vi "enable_channels.vi"(5 "channel":i32[](array[numeric]), 6 "celay":i32[](array[numeric]), 7 "vclip":i32[](array[numeric]), 8 "error in":errorcluster, 9 "vatt":i32[](array[numeric]), 10 "id_in":i32, 11 "connection ID":refnum<k5>) -> (0 "error out":errorcluster, 1 "id_out":i32, 3 "connection ID out":refnum<k5>)   [LabVIEW 2009]
doc: "This VI sends a command to the Integration Board and provides the received data when necessary."
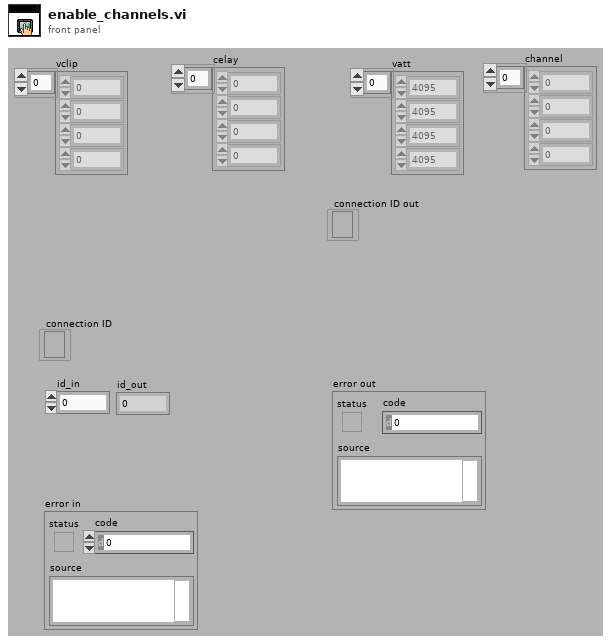
[diagram p1: front panel]
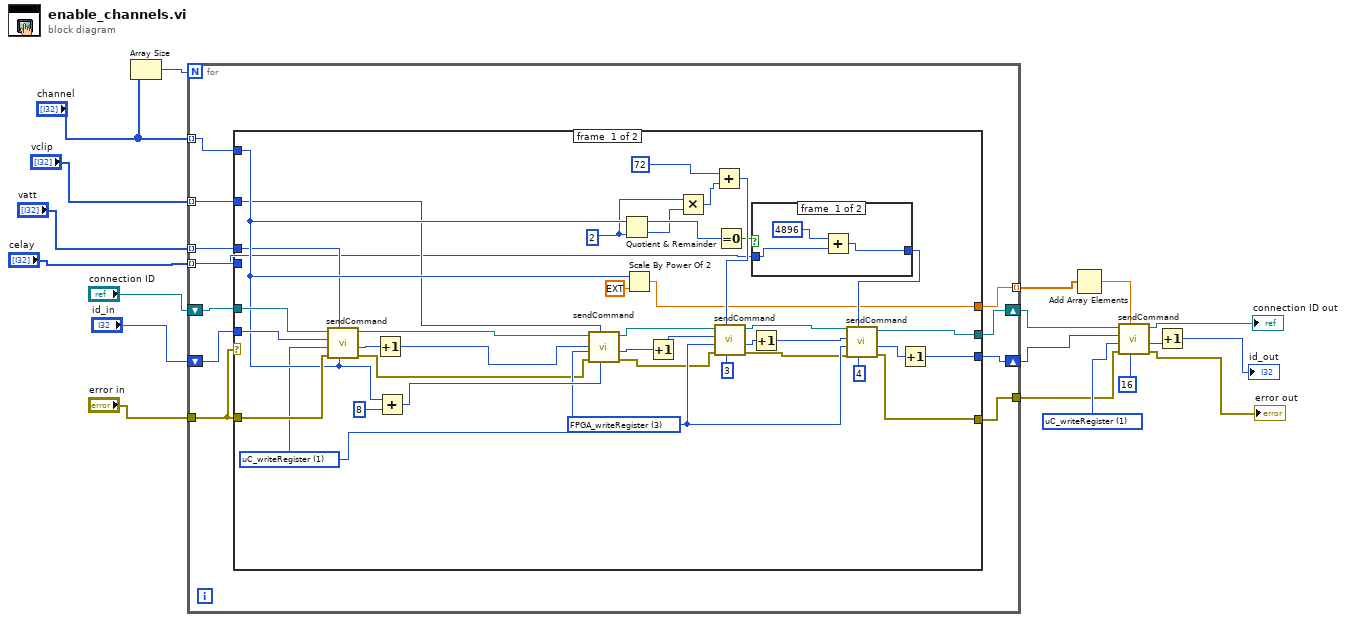
[diagram p0: block diagram]
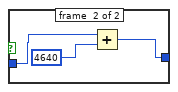
[diagram p2: hidden frame]
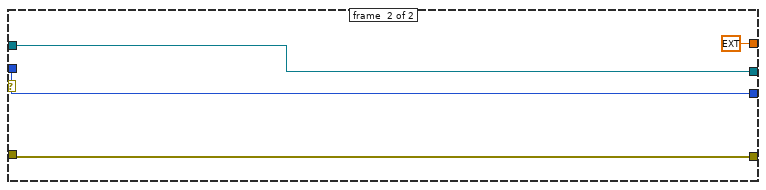
[diagram p3: hidden frame]
diagram:
  w14 = u16 1 items=["sendCommand"=9, "FPGA_writeRegister"=3, "FPGA_readRegister"=2, "uC_writeRegister"=1, "uC_readRegister"=0] ("Action")
  n1 = Array Size(array="channel") -> (size(s)=w2:i32)
  n2 = for {
    N: w2 -> [_]
    tunnel: "channel" -> [w28] mode=indexing
    tunnel: "error in" -> [w27]
    tunnel: "vatt" -> [w26] mode=indexing
    tunnel: "vclip" -> [w25] mode=indexing
    tunnel: "celay" -> [w24] mode=indexing
    tunnel: [w23] -> w10
    tunnel: [w21] -> w8 mode=indexing
    shift-right: [w22] -> w9
    shift-left: "connection ID" -> [w29]
    shift-right: [w20] -> w1
    shift-left: "id_in" -> [w30]
    n3 = case shown="No Error" w27 {
      tunnel: w30 -> [w67 w77]
      tunnel: w27 -> [w68 w78]
      tunnel: w29 -> [w69 w79]
      tunnel: [w35 w78] -> w23
      tunnel: [w60 w79] -> w22
      tunnel: w28 -> [w49 _]
      tunnel: [w55 w77] -> w20
      tunnel: w26 -> [w41 _]
      tunnel: w25 -> [w40 _]
      tunnel: w24 -> [w38 _]
      tunnel: [w31 ext 0.0] -> w21
      frame #0 {
        w39 = u16 1 items=["sendCommand"=9, "FPGA_writeRegister"=3, "FPGA_readRegister"=2, "uC_writeRegister"=1, "uC_readRegister"=0] ("Action")
        w43 = u16 2 ("y")
        w54 = u16 3 items=["sendCommand"=9, "FPGA_writeRegister"=3, "FPGA_readRegister"=2, "uC_writeRegister"=1, "uC_readRegister"=0] ("Action")
        n4 = call "sendCommand.vi"("Address"=w49, "Data"=w41, "error in"=w68, "Action"=w39, "id_in"=w67, "connection ID"=w69) -> ("error out"=w36:errorcluster, "id_out"=w65:i32, "connection ID out"=w64:refnum<k5>)  [unwired: 1 in, 2 out]
        n5 = Increment(x=w65) -> (x+1=w42:i32)
        n6 = Add(x=w49, y=u16 8) -> (x+y=w62:i32)
        n7 = call "sendCommand.vi"("Address"=w62, "Data"=w40, "error in"=w36, "Action"=w39, "id_in"=w42, "connection ID"=w64) -> ("error out"=w32:errorcluster, "id_out"=w66:i32, "connection ID out"=w34:refnum<k5>)  [unwired: 1 in, 2 out]
        n8 = Quotient & Remainder(x=w49, y=w43) -> (x-y*floor(x/y)=w46:i32, floor(x/y)=w45:i32)
        n9 = Scale By Power Of 2(n=w49, x=ext 1.0) -> (x*2^n=w31:ext)
        n10 = Increment(x=w66) -> (x+1=w33:i32)
        n11 = Multiply(x=w43, y=w45) -> (x*y=w44:i32)
        n12 = Add(x=72 ("Data"), y=w44) -> (x+y=w50:i32)
        n13 = call "sendCommand.vi"("Address"=3, "Data"=w50, "error in"=w32, "Action"=w54, "id_in"=w33, "connection ID"=w34) -> ("error out"=w37:errorcluster, "id_out"=w57:i32, "connection ID out"=w59:refnum<k5>)  [unwired: 1 in, 2 out]
        n14 = Equal To 0?(x=w46) -> (x = 0?=w48:bool)
        n15 = Increment(x=w57) -> (x+1=w58:i32)
        n16 = case shown="True" w48 {
          tunnel: [w71 w73] -> w47
          tunnel: w38 -> [w70 w74]
          frame #0 {
            n17 = Add(x=4896 ("Data"), y=w70) -> (x+y=w71:i32)
          }
          frame #1 {
            n18 = Add(x=w74, y=4640 ("Data")) -> (x+y=w73:i32)
          }
        }
        n19 = call "sendCommand.vi"("Address"=4, "Data"=w47, "error in"=w37, "Action"=w54, "id_in"=w58, "connection ID"=w59) -> ("error out"=w35:errorcluster, "id_out"=w56:i32, "connection ID out"=w60:refnum<k5>)  [unwired: 1 in, 2 out]
        n20 = Increment(x=w56) -> (x+1=w55:i32)
      }
      frame #1 {
      }
    }
  }
  n21 = Add Array Elements(numeric array=w8) -> (sum=w7:ext)
  n22 = call "sendCommand.vi"("Address"=16, "Data"=w7, "error in"=w10, "Action"=w14, "id_in"=w1, "connection ID"=w9) -> ("error out"=→"error out":errorcluster, "id_out"=w16:i32, "connection ID out"=→"connection ID out":refnum<k5>)  [unwired: 1 in, 2 out]
  n23 = Increment(x=w16) -> (x+1=→"id_out":i32)
